vi "Open Project.vi"(8 "error in (no error)":errorcluster, 9 "project index":i32, 10 "name or relative path":string, 11 "User folder Path":path) -> (0 "error out":errorcluster, 1 "Input Cluster":T1={"Project Info"={"Project Name"="New Project", "City"="", "State"="", "Notes"=""}, "Basic Inputs"={"Q.Plant"=0.05, "C.CoagDoseMax"=0.01, "C.CoagStock"=0.01, "Ti.CoagStock"=0.0015, "EN.DrillSeries"=enum."English", "EN.TubeSeries"=enum."English", "N.SedTanks"=10.0, "N.SedBaysEst"=120.0, "W.SedPlate"=0.04, "L.SedPlateSheet"=0.0, "T.SedPlate"=388800000.0, "T.PlantWall"=0.03, "H.FlocOption"=0.02, "T.FlocBaffleRigidH"=0.03, "T.ConcreteMin"=0.3, "T.SedWeir"=0.04, "T.FlocBaffleRigidV"=72000.0}} {"Basic Inputs"."T.FlocBaffleRigidV" min=0.0 max=0.2 step=0.001 format="%#.1f"; "Basic Inputs"."T.SedWeir" min=0.001 max=0.2 step=0.001 format="%#.1f"; "Basic Inputs"."T.SedPlate" min=0.001 max=0.05 step=0.001 format="%#.1f"; "Basic Inputs"."T.FlocBaffleRigidH" min=0.0 max=0.2 step=0.001 format="%#.1f"; "Basic Inputs"."T.ConcreteMin" min=0.005 max=0.2 step=0.001 format="%#.1f"; "Basic Inputs"."L.SedPlateSheet" min=0.3 max=8.0 step=0.01 format="%#.1f"; "Basic Inputs"."N.SedBaysEst" min=1.0 max=20.0 step=1.0 format="%#.0f"; "Basic Inputs"."N.SedTanks" min=1.0 max=20.0 step=1.0 format="%#.0f"; "Basic Inputs"."Ti.CoagStock" min=43200.0 max=360000.0 step=3600.0 format="%#.1f"; "Basic Inputs"."H.FlocOption" min=0.5 max=4.0 step=0.01 format="%#.2f"; "Basic Inputs"."C.CoagStock" min=50.0 max=500.0 step=1.0 format="%#.0f"; "Basic Inputs"."C.CoagDoseMax" min=0.03 max=0.2 step=0.005 format="%#.0f"; "Basic Inputs"."Q.Plant" min=0.001 max=0.2 step=0.0001 format="%#.1f"; "Basic Inputs"."T.PlantWall" min=0.05 max=0.5 step=0.001 format="%#.1f"; "Basic Inputs"."W.SedPlate" min=0.5 max=3.0 step=0.001 format="%#.1f"}, 3 "Project Folder":path, 6 "File List":string[](array[string]))   [LabVIEW 2015]
uses:
  Input Cluster.ctl
  Project inputs.ctl
  Basic Inputs.ctl
  AguaClara Library.lvlib
panel:
  out "data":cluster{"Label.Text":string, "Value":variant}[](array[cluster])
  out "data file path":path
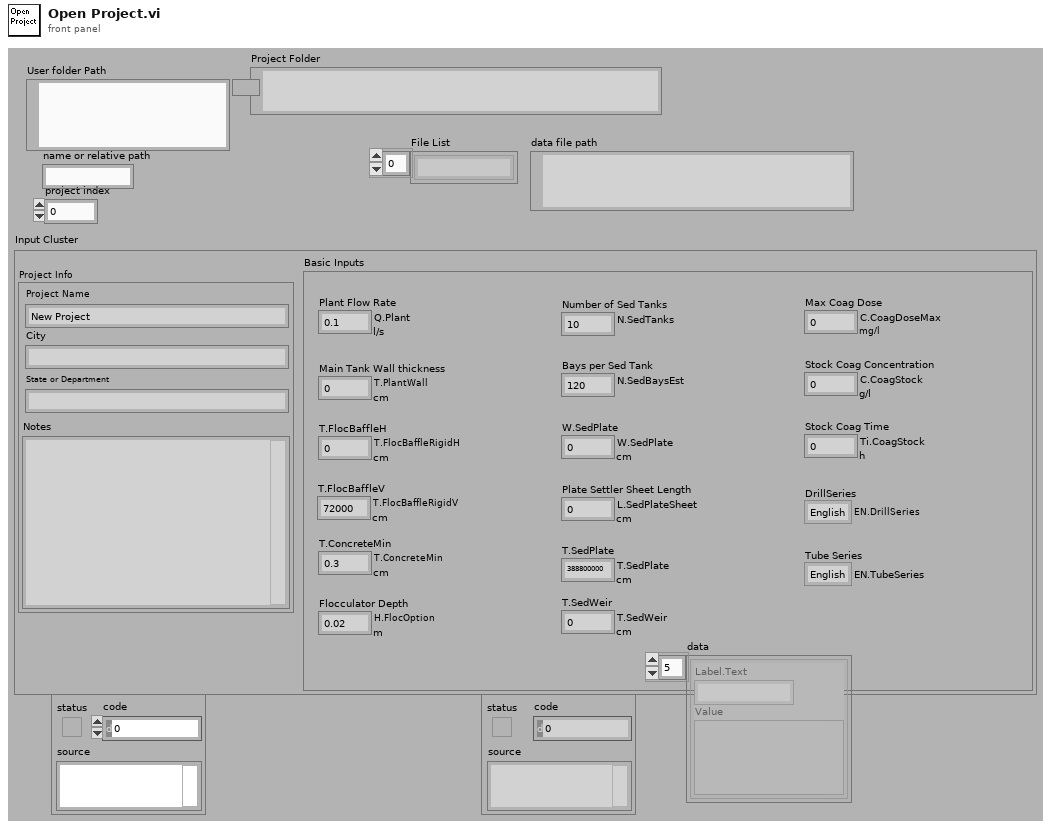
[diagram p1: front panel]
types:
  T1 = typedef "Input Cluster.ctl" = cluster{"Project Info":T2, "Basic Inputs":T3}
  T2 = typedef "AguaClara Library.lvlib/Project inputs.ctl" = cluster{"Project Name":string, "City":string, "State":string, "Notes":string}
  T3 = typedef "AguaClara Library.lvlib/Basic Inputs.ctl" = cluster{"Q.Plant":dbl[unit], "C.CoagDoseMax":dbl[unit], "C.CoagStock":dbl[unit], "Ti.CoagStock":dbl[unit], "EN.DrillSeries":enum16{"English", "Metric"}, "EN.TubeSeries":enum16{"English", "Metric"}, "N.SedTanks":dbl, "N.SedBaysEst":dbl, "W.SedPlate":dbl[unit], "L.SedPlateSheet":dbl[unit], "T.SedPlate":dbl[unit], "T.PlantWall":dbl[unit], "H.FlocOption":dbl[unit], "T.FlocBaffleRigidH":dbl[unit], "T.ConcreteMin":dbl[unit], "T.SedWeir":dbl[unit], "T.FlocBaffleRigidV":dbl[unit]}
  T4 = enum16{"open", "replace", "create", "open or create", "replace or create", "replace or create with confirmation"}
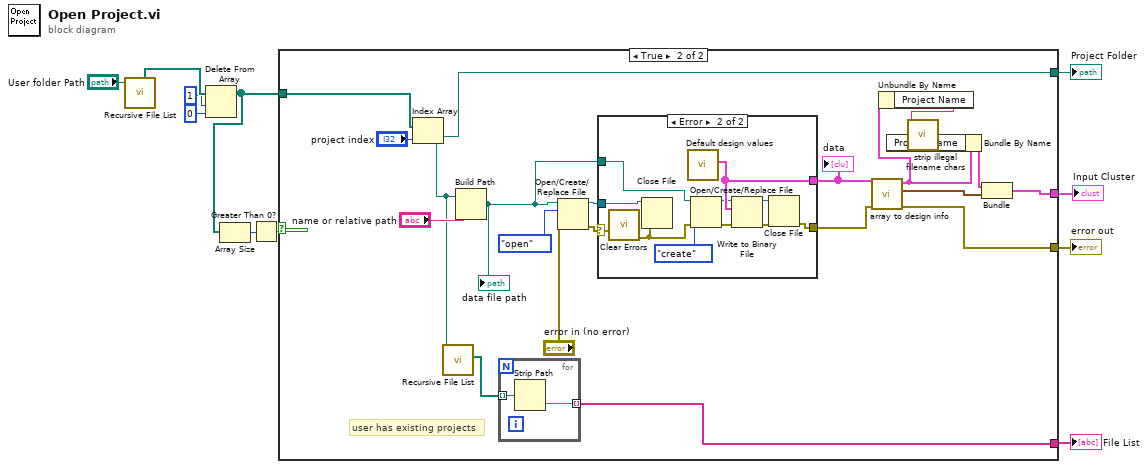
[diagram p0: block diagram]
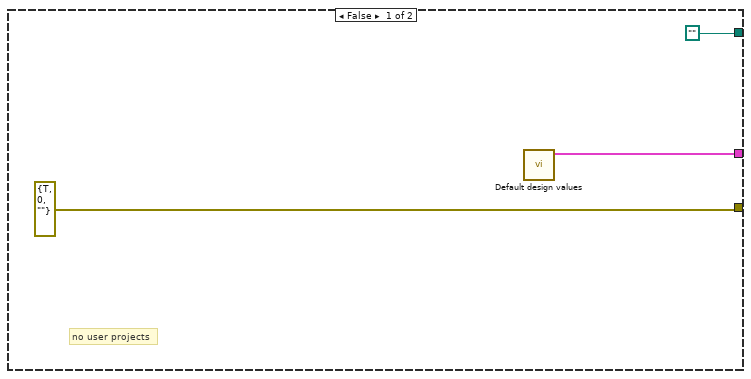
[diagram p2: hidden frame]
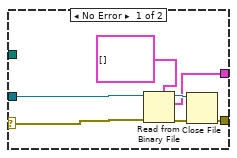
[diagram p3: hidden frame]
diagram:
  n1 = call <vilib>:"Recursive File List.vi"("Folder Path"="User folder Path") -> ("All Folders"=w10:path[])  [unwired: 6 in, 4 out]
  n2 = Delete From Array(array=w10, length=1, index=0) -> (array with subset deleted=w7:path[])  [unwired: 1 out]
  n3 = Array Size(array=w7) -> (size(s)=w6:i32)
  n4 = Greater Than 0?(x=w6) -> (x > 0?=w5:bool)
  n5 = case shown="True" w5 {
    tunnel: w7 -> [_ w30]
    tunnel: [_ w26] -> w3
    tunnel: [path "" w28] -> w4
    tunnel: [errorcluster {"status"=TRUE, "code"=0, "source"=""} ("error out") w22] -> w2
    tunnel: [w12 w24] -> w1
    frame False {
      # "no user projects"
      n6 = call "Default design values.vi"() -> ("Input Cluster"=w12:T1)  [unwired: 9 in, 2 out]
    }
    frame True {
      # "user has existing projects"
      n7 = Index Array(array=w30, index="project index") -> (element=w28:path)
      n8 = call <vilib>:"Recursive File List.vi"("Folder Path"=w28) -> ("All Files in Dir"=w29:path[])  [unwired: 6 in, 4 out]
      n9 = Build Path(base path=w28, name or relative path="name or relative path") -> (appended path=w19:path)
      "data file path" <- w19
      n10 = for {
        tunnel: w29 -> [w54] mode=indexing
        tunnel: [w53] -> w26 mode=indexing
        n11 = Strip Path(path=w54) -> (name=w53:string)  [unwired: 1 out]
      }
      n12 = Open/Create/Replace File(file path (use dialog)=w19, error in="error in (no error)", operation (0:open)=T4."open") -> (refnum out=w32:refnum<file>, error out=w21:errorcluster)  [unwired: 3 in, 1 out]
      n13 = case shown="Error" w21 {
        selector: w21 -> [w35 w52]
        tunnel: w32 -> [w41 w51]
        tunnel: [w38 w48] -> w27
        tunnel: [w37 w44] -> w23
        tunnel: w19 -> [_ w43]
        frame No Error {
          n14 = Read from Binary File(5:cluster{"Label.Text":string, "Value":variant}[] [] ("data"), 8:w35, 11:w41) -> (0:w39:errorcluster, 2:w38:cluster{"Label.Text":string, "Value":variant}[], 3:w40:refnum<file>)  [unwired: 3 in, 1 out]
          n15 = Close File(refnum=w40, error in=w39) -> (error out=w37:errorcluster)  [unwired: 1 out]
        }
        frame Error {
          n16 = call <vilib>:"Clear Errors.vi"("error in (no error)"=w52) -> ("error out"=w42:errorcluster)  [unwired: 5 in, 1 out]
          n17 = Close File(refnum=w51, error in=w42) -> ()  [unwired: 2 out]
          n18 = call "Default design values.vi"() -> ("Array to save"=w48:cluster{"Label.Text":string, "Value":variant}[])  [unwired: 9 in, 2 out]
          n19 = Open/Create/Replace File(file path (use dialog)=w43, error in=w42, operation (0:open)=T4."create") -> (refnum out=w47:refnum<file>, error out=w49:errorcluster)  [unwired: 3 in, 1 out]
          n20 = Write to Binary File(file (use dialog)=w47, data=w48, error in=w49) -> (refnum out=w45:refnum<file>, error out=w46:errorcluster)  [unwired: 3 in, 1 out]
          n21 = Close File(refnum=w45, error in=w46) -> (error out=w44:errorcluster)  [unwired: 1 out]
        }
      }
      "data" <- w27
      n22 = call "array to design info.vi"("error in (no error)"=w23, "Array from file"=w27) -> ("error out"=w22:errorcluster, "Design Inputs"=w25:T3, "Project Info"=w16:T2)  [unwired: 7 in]
      n23 = Unbundle By Name(w16) -> ("Project Name"=w18:string)
      n24 = call "strip illegal filename chars.vi"("string in"=w18) -> ("string out"=w17:string)  [unwired: 10 in]
      n25 = Bundle By Name(cluster=w16, "Project Name"=w17) -> (w15:T2)
      n26 = Bundle("Project Info"=w15, "Design Inputs"=w25) -> (w24:cluster{"Project Info":T2, "Design Inputs":T3})  [unwired: 1 in]
    }
  }
  "Project Folder" <- w4
  "File List" <- w3
  "error out" <- w2
  "Input Cluster" <- w1
